vi "Fire User Event - Update Display.vi"(8 "error in (no error)":errorcluster, 10 "event data":string, 11 "Update Display":refnum<user-event>) -> (0 "error out":errorcluster)   [LabVIEW 2018]
doc: "Send the Stop event to stop the Event Handling Loop."
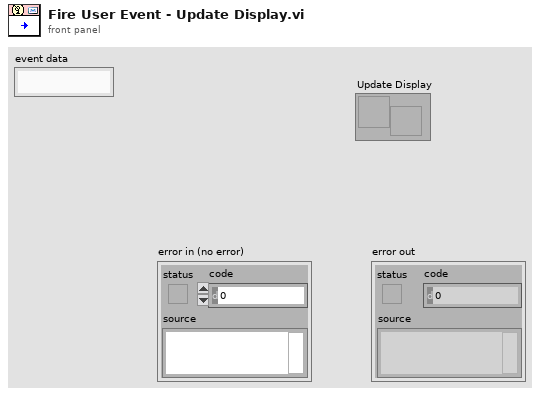
[diagram p1: front panel]
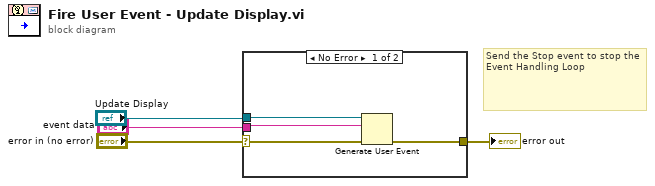
[diagram p0: block diagram]
diagram:
  # "Send the Stop event to stop the Event Handling Loop"
  n1 = case shown="No Error" "error in (no error)" {
    selector: "error in (no error)" -> [w6 w9]
    tunnel: [w8 w9] -> w4
    tunnel: "Update Display" -> [w7 _]
    tunnel: "event data" -> [w5 _]
    frame No Error {
      n2 = Generate User Event(user event=w7, event data cluster=w5, error in=w6) -> (error out=w8:errorcluster)  [unwired: 1 in, 1 out]
    }
    frame Error {
    }
  }
  "error out" <- w4
